vi "Write Static Overlays.vi"(8 "error in (no error)":errorcluster, 10 "Static Overlays":refnum<class "Static Overlay.lvclass">[](array[class]), 11 "HIJ Vision Display in":refnum<class "HIJ Vision Display.lvclass">) -> (0 "error out":errorcluster, 3 "HIJ Vision Display out":refnum<class "HIJ Vision Display.lvclass">)   [LabVIEW 2014, in "HIJ Vision Display.lvlib" / "HIJ Vision Display.lvclass"]
uses:
  HIJ Vision Display.lvclass
  Analyze/Results and Overlays/Static Overlay/Static Overlay.lvclass
  HIJ Vision Display.lvclass/HIJ Vision Display.ctl
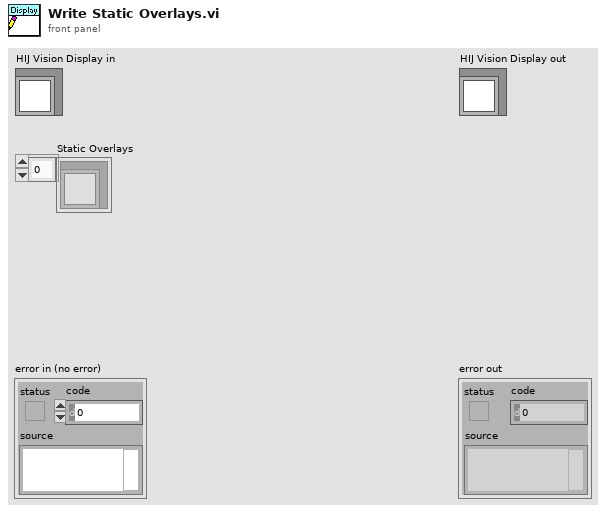
[diagram p1: front panel]
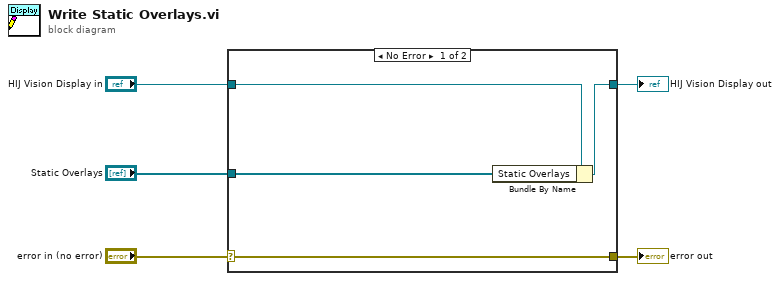
[diagram p0: block diagram]
diagram:
  n1 = case shown="No Error" "error in (no error)" {
    selector: "error in (no error)" -> [w9 w10]
    tunnel: [w9 w10] -> w4
    tunnel: [w6 w11] -> w2
    tunnel: "HIJ Vision Display in" -> [w7 w11]
    tunnel: "Static Overlays" -> [w8 _]
    frame No Error {
      n2 = Bundle By Name(cluster=w7, "Static Overlays"=w8) -> (w6:refnum<class "HIJ Vision Display.lvclass">)
    }
    frame Error {
    }
  }
  "error out" <- w4
  "HIJ Vision Display out" <- w2
